vi "CRYTest Duplicate Channels.vi"(10 "Channel Info":T1[](array[typedef]) {"Coupling" items=["Default"=-1, "RSE"=10083, "NRSE"=10078, "Differential"=10106, "Pseudodifferential"=12529]; "term config" items=["Default"=-1, "RSE"=10083, "NRSE"=10078, "Differential"=10106, "Pseudodifferential"=12529]; "Anti-aliasing Factor (%fs)" format="%.2f"}, 11 "Channel Name":string) -> (2 "index of element":i32, 3 "Exist Flag":bool)   [LabVIEW 2013]
uses:
  Typedef Control/CRYHardware Channel Info.ctl
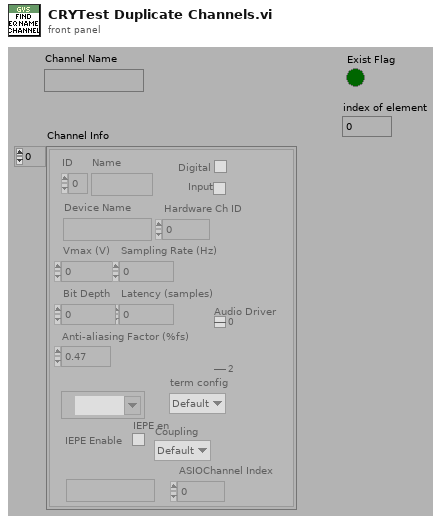
[diagram p1: front panel]
types:
  T1 = typedef "CRYHardware Channel Info.ctl" = cluster{"ID":i32, "Name":string, "Digital":bool, "Input":bool, "Device Name":string, "Hardware Ch ID":u8, "Vmax (V)":dbl, "Latency (samples)":dbl, "Sampling Rate (Hz)":u32, "Bit Depth":u32, "Anti-aliasing Factor (%fs)":sgl, "DAQmx Channel":tag, "term config":i32, "Coupling":i32, "IEPE en":bool, "ASIOChannel Name":string, "Audio Driver":u16, "ASIOChannel Index":u8}
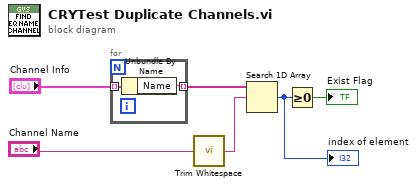
[diagram p0: block diagram]
diagram:
  n1 = for {
    tunnel: "Channel Info" -> [w8] mode=indexing
    tunnel: [w7] -> w4 mode=indexing
    n2 = Unbundle By Name(w8) -> ("Name"=w7:string)
  }
  n3 = call <vilib>:"Trim Whitespace.vi"("string"="Channel Name") -> ("trimmed string"=w3:string)  [unwired: 1 in]
  n4 = Search 1D Array(1D array=w4, element=w3) -> (index of element=w2:i32)  [unwired: 1 out]
  "index of element" <- w2
  n5 = Greater Or Equal To 0?(x=w2) -> (x >= 0?=→"Exist Flag":bool)
